vi "Track and SPCM New 2.vi"(0 "X Parameters":T2={"Number of X Steps"=200, "Max X (V)"=1.0, "Min X (V)"=-1.0}, 1 "X Pos":dbl=125.0, 2 "Scan Interval (minutes)":dbl=2.0, 3 "Y pos":dbl=47.0, 5 "Y Parameters":T1={"Number of Y Steps"=200, "Max Y (V)"=1.0, "Min Y (V)"=-1.0}, 7 "Z interval (min)":dbl=10.0, 9 "RS232 settings":cluster{"Portnumber":i32, "Baudrate":u16}={"Portnumber"=6, "Baudrate"=5} {"Portnumber" items=["COM1", "COM2", "COM3", "COM4", "COM5", "COM6", "COM7", "COM8", "COM9", "COM10", "COM11", "COM12", "COM13", "COM14", "COM15", "COM16", "COM17", "COM18", "COM19", "COM20", "COM21", "COM22", "COM23", "COM24", "COM25", "COM26", "COM27", "COM28", "COM29", "COM30"]; "Baudrate" items=["9600", "14400", "19200", "38400", "57600", "115200"]}, 11 "Z Pos":dbl=53.4, 12 "SPCM File Path":path=path "C:/Users/Ouyang Group/Documents/Data/6-11-15/ND 40 Au DC PVB med power -1to1 Scan 5 x125 y47.spc", 13 "Collection Time (hours)":dbl=3.0, 14 "Tracking Data File Path":path=path "C:/Users/Ouyang Group/Documents/Data/6-11-15/ND 40 Au DC PVB med power -1to1 Scan 5 x125 y47 position tracking.txt") -> (4 "X Position":dbl, 6 "Y Position":dbl, 8 "Z Position":dbl)   [LabVIEW 2012]
uses:
  SPCM files/Global FIFO variabls.vi
  <vilib>/Utility/file.llb/Write To Spreadsheet File (DBL).vi
panel:
  out "Intensity":cluster{timestamp[], dbl[]}(graph)
  out "Z Position":cluster{timestamp[], dbl[]}(graph)
  out "Y Position":cluster{timestamp[], dbl[]}(graph)
  out "X Position":cluster{timestamp[], dbl[]}(graph)
  in  "stop":bool
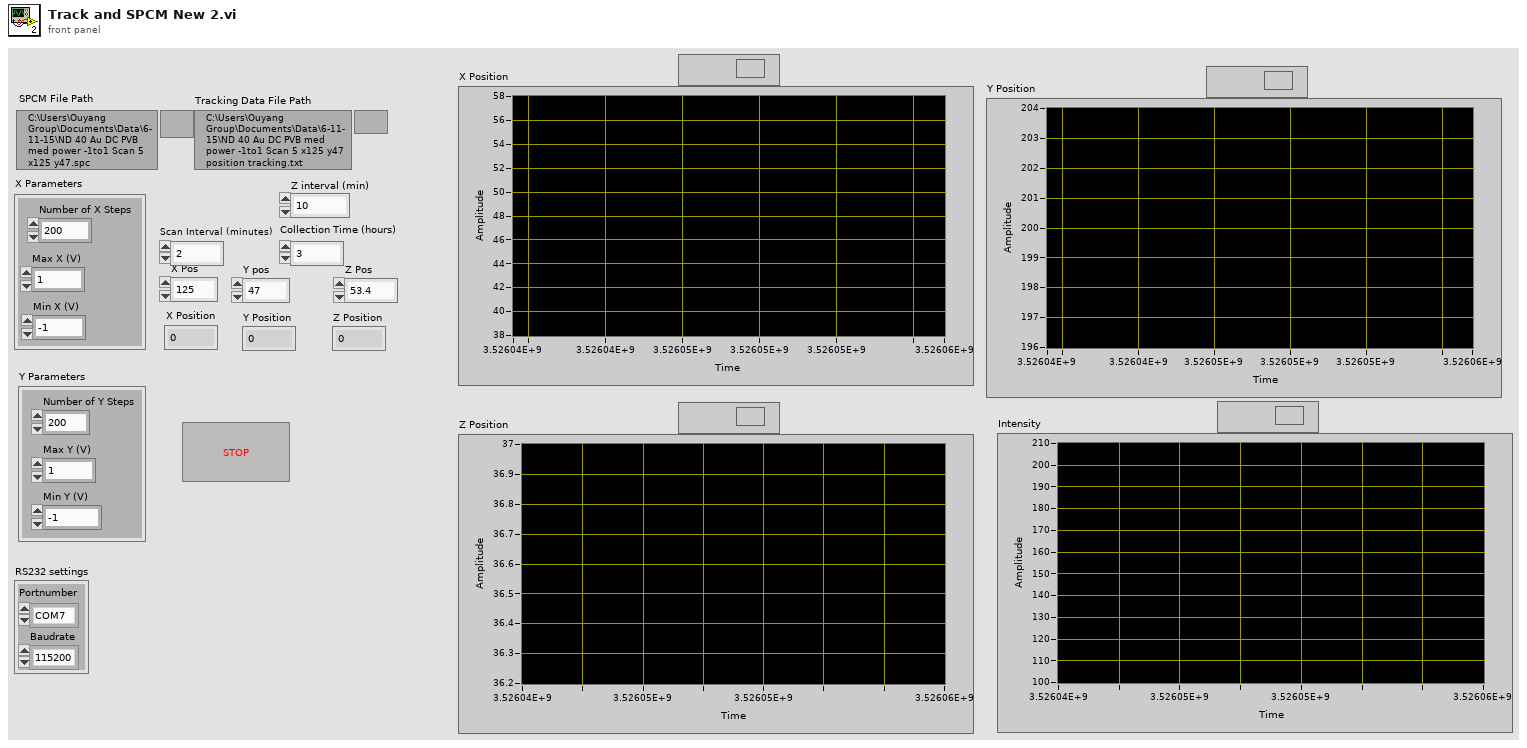
[diagram p1: front panel]
types:
  T1 = cluster{"Number of Y Steps":i32, "Max Y (V)":dbl, "Min Y (V)":dbl}
  T2 = cluster{"Number of X Steps":i32, "Max X (V)":dbl, "Min X (V)":dbl}
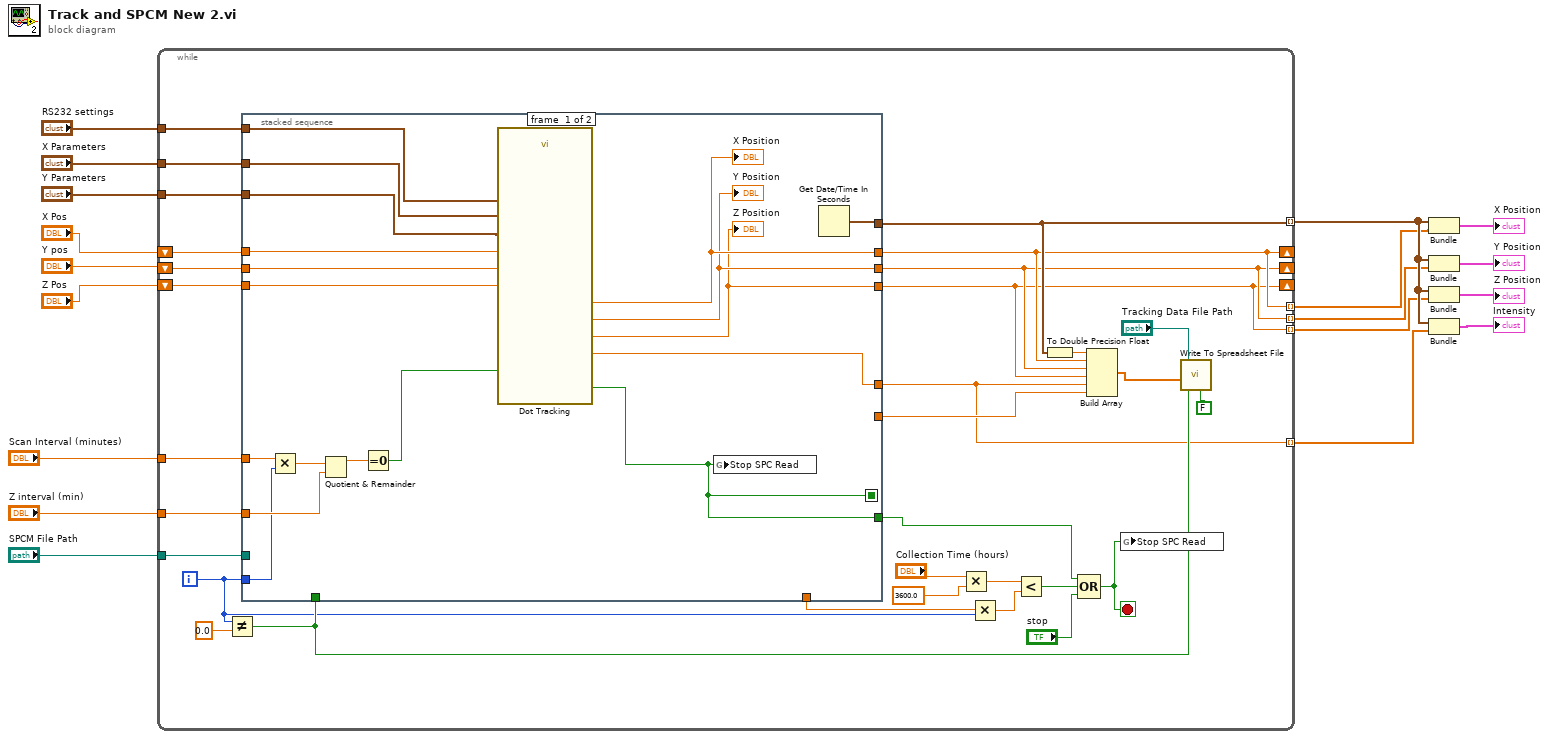
[diagram p0: block diagram]
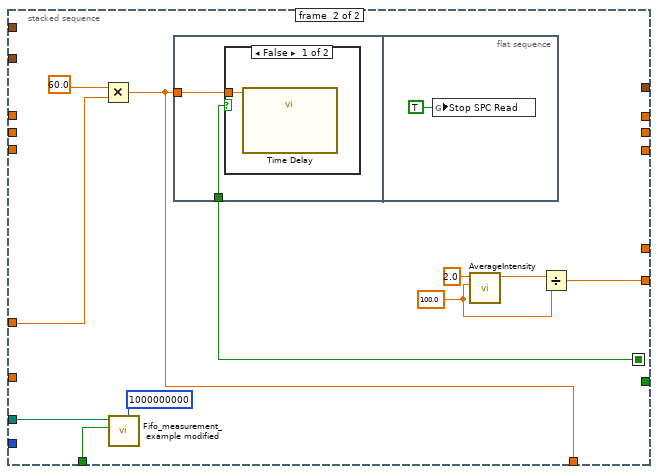
[diagram p2: hidden frame]
diagram:
  n1 = while {
    shift-right: [w21] -> _
    shift-left: "X Pos" -> [w37]
    shift-right: [w20] -> _
    shift-left: "Y pos" -> [w36]
    shift-right: [w19] -> _
    shift-left: "Z Pos" -> [w35]
    tunnel: "Scan Interval (minutes)" -> [w42]
    tunnel: "Z interval (min)" -> [w41]
    tunnel: "RS232 settings" -> [w40]
    tunnel: "X Parameters" -> [w39]
    tunnel: "Y Parameters" -> [w38]
    tunnel: "SPCM File Path" -> [w32]
    tunnel: [w23] -> w8 mode=indexing
    tunnel: [w22] -> w9 mode=indexing
    tunnel: [w21] -> w3 mode=indexing
    tunnel: [w20] -> w2 mode=indexing
    tunnel: [w19] -> w1 mode=indexing
    i -> [w34]
    stop <- w27 stop-if-true
    n2 = Not Equal?(x=w34, y=0.0 ("x")) -> (x != y?=w43:bool)
    n3 = stacked-sequence {
      seq-local: [w67 _] -> [_ w76]
      tunnel: w43 -> [_ w78]
      tunnel: [w52 _] -> w22
      tunnel: [w67 _] -> w29
      tunnel: w42 -> [w64 w70]
      tunnel: w41 -> [w62 _]
      tunnel: w40 -> [w59 _]
      tunnel: w39 -> [w60 _]
      tunnel: w38 -> [w61 _]
      tunnel: w37 -> [w58 _]
      tunnel: w36 -> [w57 _]
      tunnel: w35 -> [w56 _]
      tunnel: [w55 _] -> w21
      tunnel: [w54 _] -> w20
      tunnel: [w53 _] -> w19
      tunnel: w34 -> [w51 _]
      tunnel: w32 -> [_ w72]
      tunnel: [_ w69] -> w25
      tunnel: [_ w68] -> w31
      tunnel: [w50 _] -> w23
      frame #0 {
        n4 = Multiply(x=w64, y=w51) -> (x*y=w63:dbl)
        n5 = Quotient & Remainder(x=w63, y=w62) -> (x-y*floor(x/y)=w66:dbl)  [unwired: 1 out]
        n6 = Equal To 0?(x=w66) -> (x = 0?=w65:bool)
        n7 = call "Dot Tracking.vi"("X"=w60, "Y Parameters"=w61, "RS232 settings"=w59, "X Pos"=w58, "Y pos"=w57, "Z Pos"=w56, "Z-track?"=w65) -> ("X Position"=w55:dbl, "Y Position"=w54:dbl, "Y Gauss Amplitude"=w50:dbl, "Z Position"=w53:dbl, "Gave up?"=w67:bool)  [unwired: 2 in, 2 out]
        "X Position" <- w55
        "Y Position" <- w54
        "Z Position" <- w53
        n8 = global write "Global FIFO variabls.vi" "Stop SPC Read"(w67) -> ()
        n9 = Get Date/Time In Seconds() -> (seconds since 1Jan1904=w52:timestamp)
      }
      frame #1 {
        w73 = 100.0 ("y")
        n10 = Multiply(x=60.0 ("y"), y=w70) -> (x*y=w68:dbl)
        n11 = call "Fifo_measurement_example modified.vi"("Required No of photons"=u32 1000000000, "append to file? (new file:F)"=w78, "file path (dialog if empty)"=w72) -> ()  [unwired: 2 in, 1 out]
        n12 = flat-sequence {
          tunnel: w76 -> [w80]
          tunnel: w68 -> [w79]
          frame #0 {
            n13 = case shown="False" w80 {
              tunnel: w79 -> [w81 _]
              frame False {
                n14 = call "Time Delay"("Delay Time (s)"=w81) -> ()  [unwired: 10 in, 1 out]
              }
              frame True {
              }
            }
          }
          frame #1 {
            n15 = global write "Global FIFO variabls.vi" "Stop SPC Read"(TRUE ("Stop SPC Read")) -> ()
          }
        }
        n16 = call "AverageIntensity.vi"("rate (Hz)"=w73, "Time Target (s)"=2.0) -> ("Average intensity (cts/s)"=w75:dbl)  [unwired: 8 in, 1 out]
        n17 = Divide(x=w75, y=w73) -> (x/y=w69:dbl)
      }
    }
    n18 = Multiply(x="Collection Time (hours)", y=3600.0) -> (x*y=w44:dbl)
    n19 = Multiply(x=w31, y=w34) -> (x*y=w45:dbl)
    n20 = Less?(x=w44, y=w45) -> (x < y?=w30:bool)
    n21 = To Double Precision Float(number=w22) -> (double precision float=w26:dbl)
    n22 = Compound Arithmetic op=OR(w29, w30, "stop") -> (w27:bool)
    n23 = Build Array(w26, w21, w20, w19, w23, w25) -> (w24:dbl[])
    n24 = global write "Global FIFO variabls.vi" "Stop SPC Read"(w27) -> ()
    n25 = call-poly <vilib>:"Write To Spreadsheet File.vi"("transpose? (no:F)"=FALSE, "append to file? (new file:F)"=w43, "1D data"=w24, "file path (dialog if empty)"="Tracking Data File Path") -> ()  [unwired: 4 in, 1 out]
  }
  n26 = Bundle(w9, w3) -> (→"X Position":cluster{timestamp[], dbl[]})  [unwired: 1 in]
  n27 = Bundle(w9, w2) -> (→"Y Position":cluster{timestamp[], dbl[]})  [unwired: 1 in]
  n28 = Bundle(w9, w1) -> (→"Z Position":cluster{timestamp[], dbl[]})  [unwired: 1 in]
  n29 = Bundle(w9, w8) -> (→"Intensity":cluster{timestamp[], dbl[]})  [unwired: 1 in]
